vi "GEOM_Cleanup0amps.vi"(10 "sorted amplifiers":T1[](array[typedef]) {"fliped" items=["none", "horizontal", "vertical"]; "type" items=["LL", "LR", "UL", "UR"]}) -> (2 "amps out":T1[](array[typedef]) {"fliped" items=["none", "horizontal", "vertical"]; "type" items=["LL", "LR", "UL", "UR"]})   [LabVIEW 2016]
uses:
  GEOM_Amplifier.ctl
  GEOM_AmpType.ctl
  GEOM_ROI.ctl
  GEOM_Coords.ctl
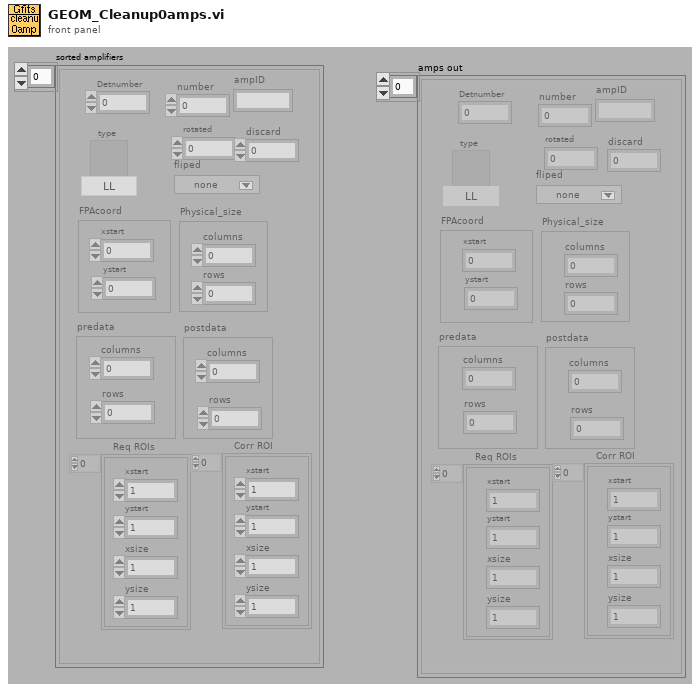
[diagram p1: front panel]
types:
  T1 = typedef "GEOM_Amplifier.ctl" = cluster{"number":i32, "type":T2, "rotated":i16, "fliped":u16, "FPAcoord":cluster{"xstart":i32, "ystart":i32}, "Physical_size":cluster{"columns":i32, "rows":i32}, "predata":cluster{"columns":i32, "rows":i32}, "postdata":cluster{"columns":i32, "rows":i32}, "Req ROIs":T3, "Corr ROI":T3, "Detnumber":i32, "ampID":string, "discard":i32}
  T2 = typedef "GEOM_AmpType.ctl" = u16
  T3 = typedef "GEOM_ROI.ctl" = T4[]
  T4 = typedef "GEOM_Coords.ctl" = cluster{"xstart":u32, "ystart":u32, "xsize":u32, "ysize":u32}
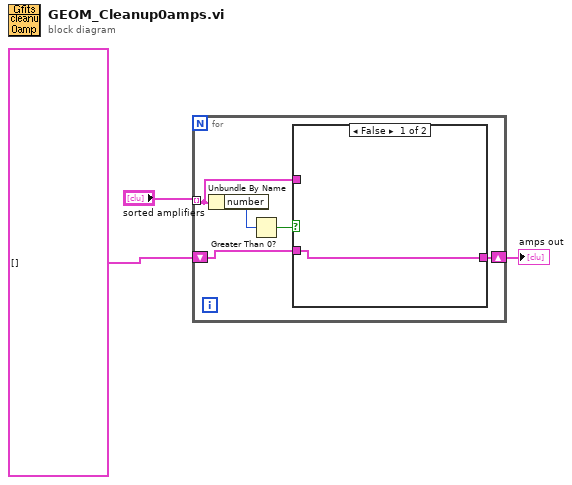
[diagram p0: block diagram]
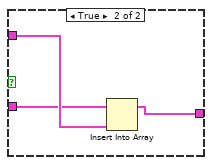
[diagram p2: hidden frame]
diagram:
  n1 = for {
    tunnel: "sorted amplifiers" -> [w6] mode=indexing
    shift-right: [w5] -> w1
    shift-left: T1[] [] -> [w4]
    n2 = Unbundle By Name(w6) -> ("number"=w8:i32)
    n3 = Greater Than 0?(x=w8) -> (x > 0?=w7:bool)
    n4 = case shown="False" w7 {
      tunnel: w6 -> [_ w12]
      tunnel: [w9 w11] -> w5
      tunnel: w4 -> [w9 w10]
      frame False {
      }
      frame True {
        n5 = Insert Into Array(array=w10, new element=w12) -> (w11:T1[])  [unwired: 1 in]
      }
    }
  }
  "amps out" <- w1
